vi "eat.vi"(0 "reference in":refnum<class "Child2.lvclass">, 5 "error in (no error)":errorcluster) -> (14 "reference out":refnum<class "Child2.lvclass">, 19 "error out":errorcluster)   [LabVIEW 2019, in "Child2.lvclass"]
uses:
  Child2.lvclass
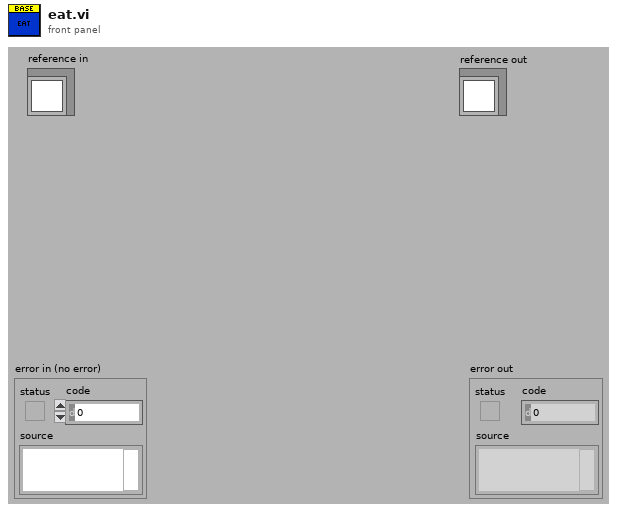
[diagram p1: front panel]
types:
  T1 = typedef "Child2.lvclass/ObjectAttributes.ctl" = cluster{"Attribute1":dbl}
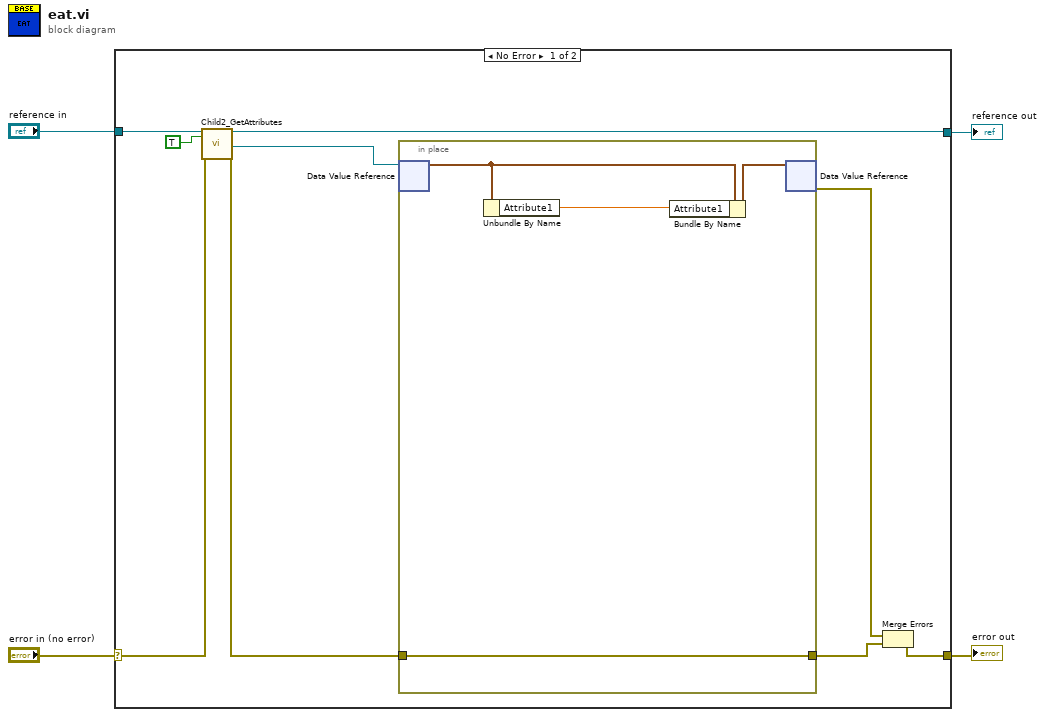
[diagram p0: block diagram]
diagram:
  n1 = case shown="No Error" "error in (no error)" {
    selector: "error in (no error)" -> [w9 w19]
    tunnel: [w12 w19] -> w3
    tunnel: [w10 w18] -> w1
    tunnel: "reference in" -> [w11 w18]
    frame No Error {
      n2 = call "Child2_GetAttributes.vi"("reference in"=w11, "OnlyGetDvrReference(False)"=TRUE, "error in (no error)"=w9) -> ("reference out"=w10:refnum<class "Child2.lvclass">, "DataRef"=w8:refnum<data-value>, "error out"=w6:errorcluster)  [unwired: 13 in, 1 out]
      n3 = in-place {
        in-place-border: w6 -> [w16]
        in-place-border: [w16] -> w5
        n4 = in-place-dvr #1(w8) -> (w15:T1)  [unwired: 1 out]
        n5 = Unbundle By Name(w15) -> ("Attribute1"=w14:dbl)
        n6 = Bundle By Name(cluster=w15, "Attribute1"=w14) -> (w17:T1)
        n7 = in-place-dvr #1(w17) -> (w13:errorcluster)  [unwired: 1 out]
      }
      n8 = Merge Errors(w13, w5) -> (w12:errorcluster)
    }
    frame Error {
    }
  }
  "error out" <- w3
  "reference out" <- w1
